vi "FTW-Endpoint-Multipart-Ask.vi"(0 "FTW Endpoint":refnum<class "FTW-Endpoint.lvclass">, 5 "Message":T1, 7 "Read Timeout":i32=100 format="%dmsec", 9 "Write Timeout":i32 format="%dmsec", 11 "error in":errorcluster) -> (4 "FTW Endpoint out":refnum<class "FTW-Endpoint.lvclass">, 6 "Reply":T1, 8 "Read Timed out?":bool, 10 "Write Timed out?":bool, 15 "error out":errorcluster)   [LabVIEW 2013, in "FTW-Endpoint.lvclass"]
uses:
  FTW-Endpoint.lvclass
  Payload/FTW-MessagePayload.ctl
  FTW-Endpoint.lvclass/FTW-Endpoint.ctl
  Ether/FTW-Ether.lvclass
panel:
  # "Inputs"
  # "Outputs"
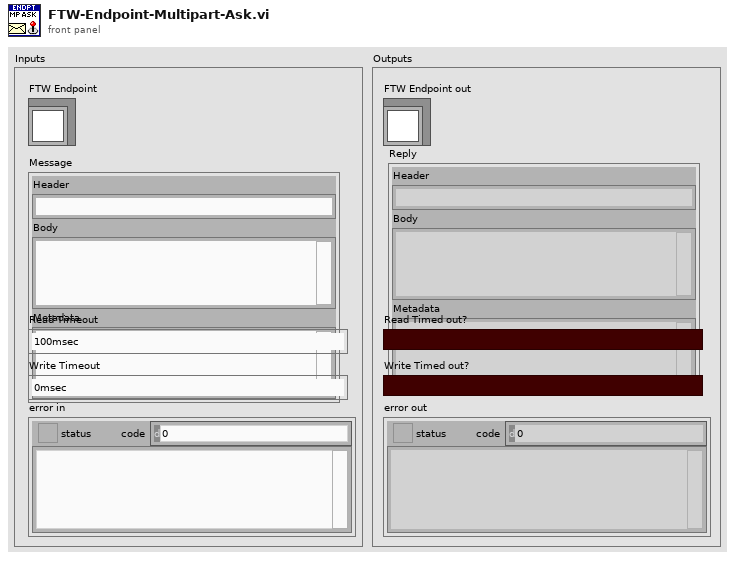
[diagram p1: front panel]
types:
  T1 = typedef "FTW-MessagePayload.ctl" = cluster{"Header":string, "Body":string, "Metadata":string}
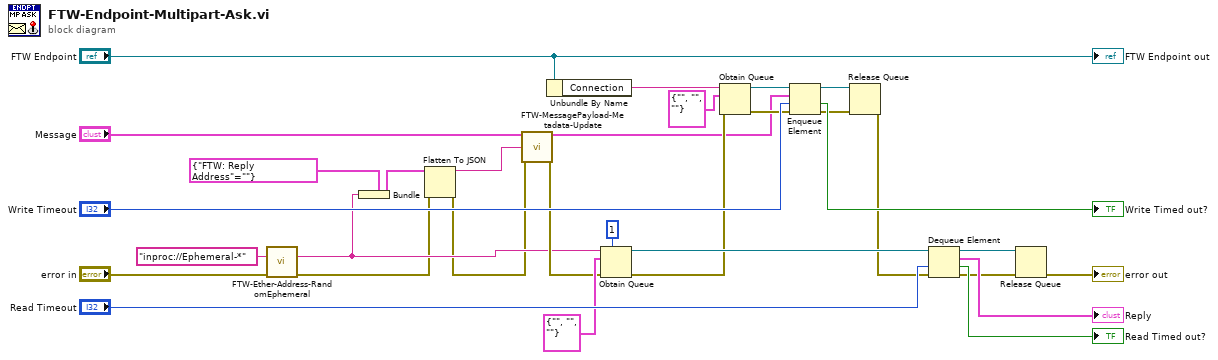
[diagram p0: block diagram]
diagram:
  n1 = call "FTW-Ether-Address-RandomEphemeral.vi"("Endpoint"="inproc://Ephemeral-*" ("Requested Ephemeral Address"), "error in"="error in") -> ("Endpoint with Replacements"=w4:string, "error out"=w2:errorcluster)  [unwired: 12 in]
  n2 = Bundle(cluster=cluster{"FTW: Reply Address":string} {"FTW: Reply Address"=""}, "FTW: Reply Address"=w4) -> (w5:cluster{"FTW: Reply Address":string})
  n3 = Flatten To JSON(anything=w5, error in (no error)=w2) -> (JSON string=w3:string, 11:w1:errorcluster)  [unwired: 1 in]
  n4 = call "FTW-MessagePayload-Metadata-Update.vi"("Message In"="Message", "Metadata"=w3, "error in"=w1) -> ("Message"=w8:T1, "error out"=w7:errorcluster)  [unwired: 11 in]
  n5 = Unbundle By Name("FTW Endpoint") -> ("Connection"=w16:string)
  n6 = Obtain Queue(max queue size (-1, unlimited)=1, name (unnamed)=w4, element data type=T1 {"Header"="", "Body"="", "Metadata"=""}, error in (no error)=w7) -> (queue out=w18:refnum<queue>, error out=w14:errorcluster)  [unwired: 1 in, 1 out]
  n7 = Obtain Queue(name (unnamed)=w16, element data type=T1 {"Header"="", "Body"="", "Metadata"=""}, error in (no error)=w14) -> (queue out=w13:refnum<queue>, error out=w15:errorcluster)  [unwired: 2 in, 1 out]
  n8 = Enqueue Element(queue=w13, element=w8, timeout in ms (-1)="Write Timeout", error in (no error)=w15) -> (queue out=w10:refnum<queue>, timed out?=→"Write Timed out?":bool, error out=w17:errorcluster)
  n9 = Release Queue(queue=w10, error in (no error)=w17) -> (error out=w11:errorcluster)  [unwired: 1 in, 2 out]
  n10 = Dequeue Element(queue=w18, timeout in ms (-1)="Read Timeout", error in (no error)=w11) -> (queue out=w23:refnum<queue>, element=→"Reply":T1, timed out?=→"Read Timed out?":bool, error out=w22:errorcluster)
  n11 = Release Queue(queue=w23, error in (no error)=w22) -> (error out=→"error out":errorcluster)  [unwired: 1 in, 2 out]
  "FTW Endpoint out" <- "FTW Endpoint"
